vi "Set Standard Bus Register Look Up Table--SubVI.vi"(8 "error in":errorcluster) -> (0 "error out":errorcluster, 3 "Standard Bus Register Look Up Table":variant)   [LabVIEW 2024, in "Watlow F4T.lvclass"]
uses:
  Watlow F4T.lvclass
  Controls/Standard Bus Register LUT Data--Cluster.ctl
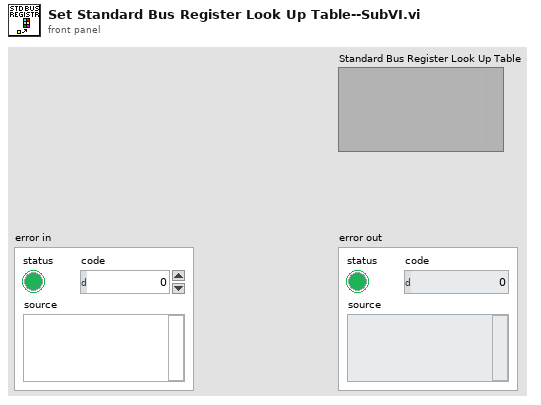
[diagram p1: front panel]
types:
  T1 = typedef "Watlow F4T.lvclass/Standard Bus Register LUT Data--Cluster.ctl" = cluster{"Parameter ID":i32, "Instance ID":i32}
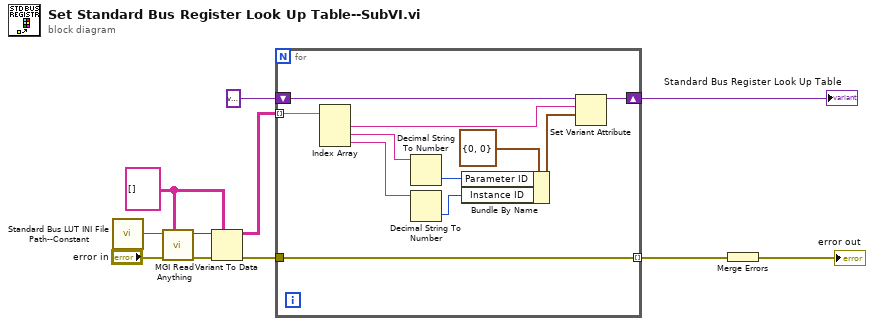
[diagram p0: block diagram]
diagram:
  w9 = string[][] []
  n1 = call "Standard Bus LUT INI File Path--Constant.vi"() -> ("Standard Bus Register LUT Path"=w2:path)  [unwired: 1 in]
  n2 = call <userlib>:"MGI Read Anything.vi"("Type of Anything"=w9, "Error In"="error in", "Path (dialog)"=w2) -> ("Error Out"=w7:errorcluster, "Anything"=w8:variant)  [unwired: 5 in, 2 out]
  n3 = Variant To Data(error in=w7, type=w9, Variant=w8) -> (data=w11:string[][], error out=w3:errorcluster)
  n4 = for {
    shift-right: [w15] -> w10
    shift-left: variant -> [w16]
    tunnel: w11 -> [w22] mode=indexing
    tunnel: [w12] -> w4 mode=indexing
    tunnel: w3 -> [w12]
    n5 = Index Array(array=w22) -> (element #1=w13:string, element #2=w21:string, element #3=w20:string)  [unwired: 3 in]
    n6 = Decimal String To Number(string=w21) -> (number=w18:i32)  [unwired: 2 in, 1 out]
    n7 = Decimal String To Number(string=w20) -> (number=w17:i32)  [unwired: 2 in, 1 out]
    n8 = Bundle By Name(cluster=T1 {"Parameter ID"=0, "Instance ID"=0} ("Parameter LUP Table Data"), "Parameter ID"=w18, "Instance ID"=w17) -> (w14:T1)
    n9 = Set Variant Attribute(Variant=w16, name=w13, value=w14) -> (Variant out=w15:variant)  [unwired: 1 in, 2 out]
  }
  "Standard Bus Register Look Up Table" <- w10
  n10 = Merge Errors(w4) -> (→"error out":errorcluster)
